vi "Shared Variable Globals.vi"() -> ()   [LabVIEW 2015, in "Shared Variable Custom Device.lvlib"]
uses:
  Shared Variable Custom Device.lvlib
panel:
  in  "Target Glyph Index":i32=47
  in  "Target Glyph":string="Glyphs\\target.png"
  in  "Folder Glyph Index":i32=46
  in  "Folder Glyph":string="Glyphs\\default Folder.png"
  in  "Shared Variable Name":string="Shared Variable Name"
  in  "Write Glyph":string="Glyphs\\write.png"
  in  "Write Glyph Index":i32=45
  in  "Read Glyph Index":i32=44
  in  "Read Glyph":string="Glyphs\\read2.png"
  in  "Boolean Glyph":string="Glyphs\\Boolean2.png"
  in  "Boolean Glyph Index":i32=43
  in  "String Glyph Index":i32=42
  in  "String Glyph":string="Glyphs\\string.png"
  in  "DBL Glyph Index":i32=41
  in  "DBL Glyph":string="Glyphs\\dbl.png"
  in  "Timeout":string="Timeout"
  in  "Status":string="Status"
  in  "Write":string="Write"
  in  "Read":string="Read"
  in  "PSP URL":string="ni.var.psp://"
  in  "Shared Variable URL":string="Shared Variable URL"
  in  "Channel Type":string="Channel Type"
  in  "Error Code":string="Error Code"
  in  "Connection Status":string="Connection Status"
  in  "IP Address":string="IP Address"
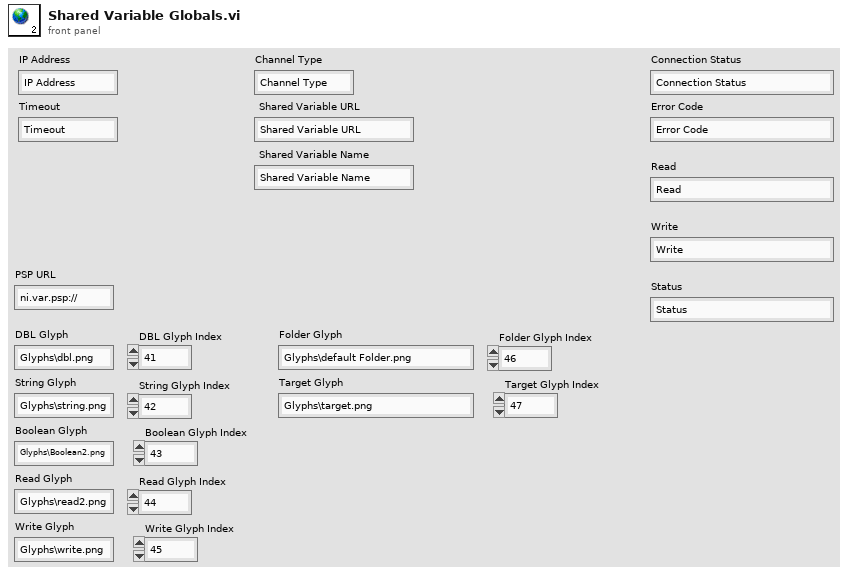
[diagram p1: front panel]
diagram:
